vi "CAN test do RIO 3 tcpip.vi"() -> ()   [LabVIEW 2014]
doc: "This example demonstrates frame streaming output using an NI-Embedded CAN for RIO interface. \n\nThis example can run against any input example, assuming you have a properly terminated CAN cable connected to two CAN ports."
uses:
  <vilib>/Platform/TimedLoop/XDataNode/XDataNode.xnode
  <vilib>/Platform/TimedLoop/XDataNode/nitl_modes.ctl
  <vilib>/Platform/TimedLoop/XDataNode/XDNodeRunTimeDep.lvlib
  <vilib>/Platform/TimedLoop/XDataNode/wakeup.ctl
  <vilib>/Platform/TimedLoop/XDataNode/timing_clust.ctl
  <resource>/objmgr/RioEmbeddedCANInterface.rc
  <vilib>/Utility/Variable/NI_VariableUtilities.lvlib
  Data Communication/Network Streams/Simple Network Streams/support/Network Stream Command.ctl
  <vilib>/RioEmbeddedCAN/RioEmbeddedCAN.llb/CANFrameControl.ctl
  <vilib>/RioEmbeddedCAN/RioEmbeddedCAN.llb/CANWaitTransmitComplete.vi
  <vilib>/NI/STM/TCP/Get Connection Reference (TCP).vi
  <vilib>/NI/STM/TCP/Write Meta Data (TCP Ref).vi
  <vilib>/NI/STM/SubVIs/MetaDataElement.ctl
  <vilib>/NI/STM/TCP/Write Message (TCP).vi
panel:
  out "error out 2":errorcluster
  in  "stop 3":bool
  out "ilosc mesag":dbl
  out "data string":string
  out "Numeric":i32
  in  "stop 2":bool
  out "Waveform Chart 5":cluster{"mean":dbl, "output 3":u16}(graph)
  out "Waveform Chart 2":cluster{"rms value":dbl, "output 2":dbl}(graph)
  in  "odczyt 2":bool=TRUE
  out "Frames 2":string[][](table) caption="Frames"
  in  "Number of Frames to Display 2":i32=15
  in  "Hexadecimal? 2":bool
  out "error out":errorcluster
  out "x != y?":bool
  out "(hi.lo)":u16
  out "x .or. y?":bool
  out "data":T1[](array[typedef]) {"type" items=["CAN Data", "CAN Remote"]; "identifier" format="%.0x"}
  in  "stop":bool
  out "Variable2":bool
  in  "CAN frame 2":T1={"identifier"=2, "extended?"=FALSE, "type"=0, "payload"=[1, 2, 3, 4, 5, 6, 7, 8]} {"type" items=["CAN Data", "CAN Remote"]; "identifier" format="%.0x"}
  in  "Stop Button":bool
  in  "Write":bool
  in  "CAN frame":T1={"identifier"=2, "extended?"=FALSE, "type"=0, "payload"=[1, 2, 3, 4, 5, 6, 7, 8]} {"type" items=["CAN Data", "CAN Remote"]; "identifier" format="%.0x"}
  in  "receive queue size":u32=50
  in  "baud rate":u32=500000
  in  "interface index":u32
  # "Overview: Demonstrates frame streaming output using an NI-Embedded CAN for RIO interface.\nInstructions: Run the VI."
  # "See VI Info <Ctrl+I> for more information on how to use this example"
  # "Interface Configuration"
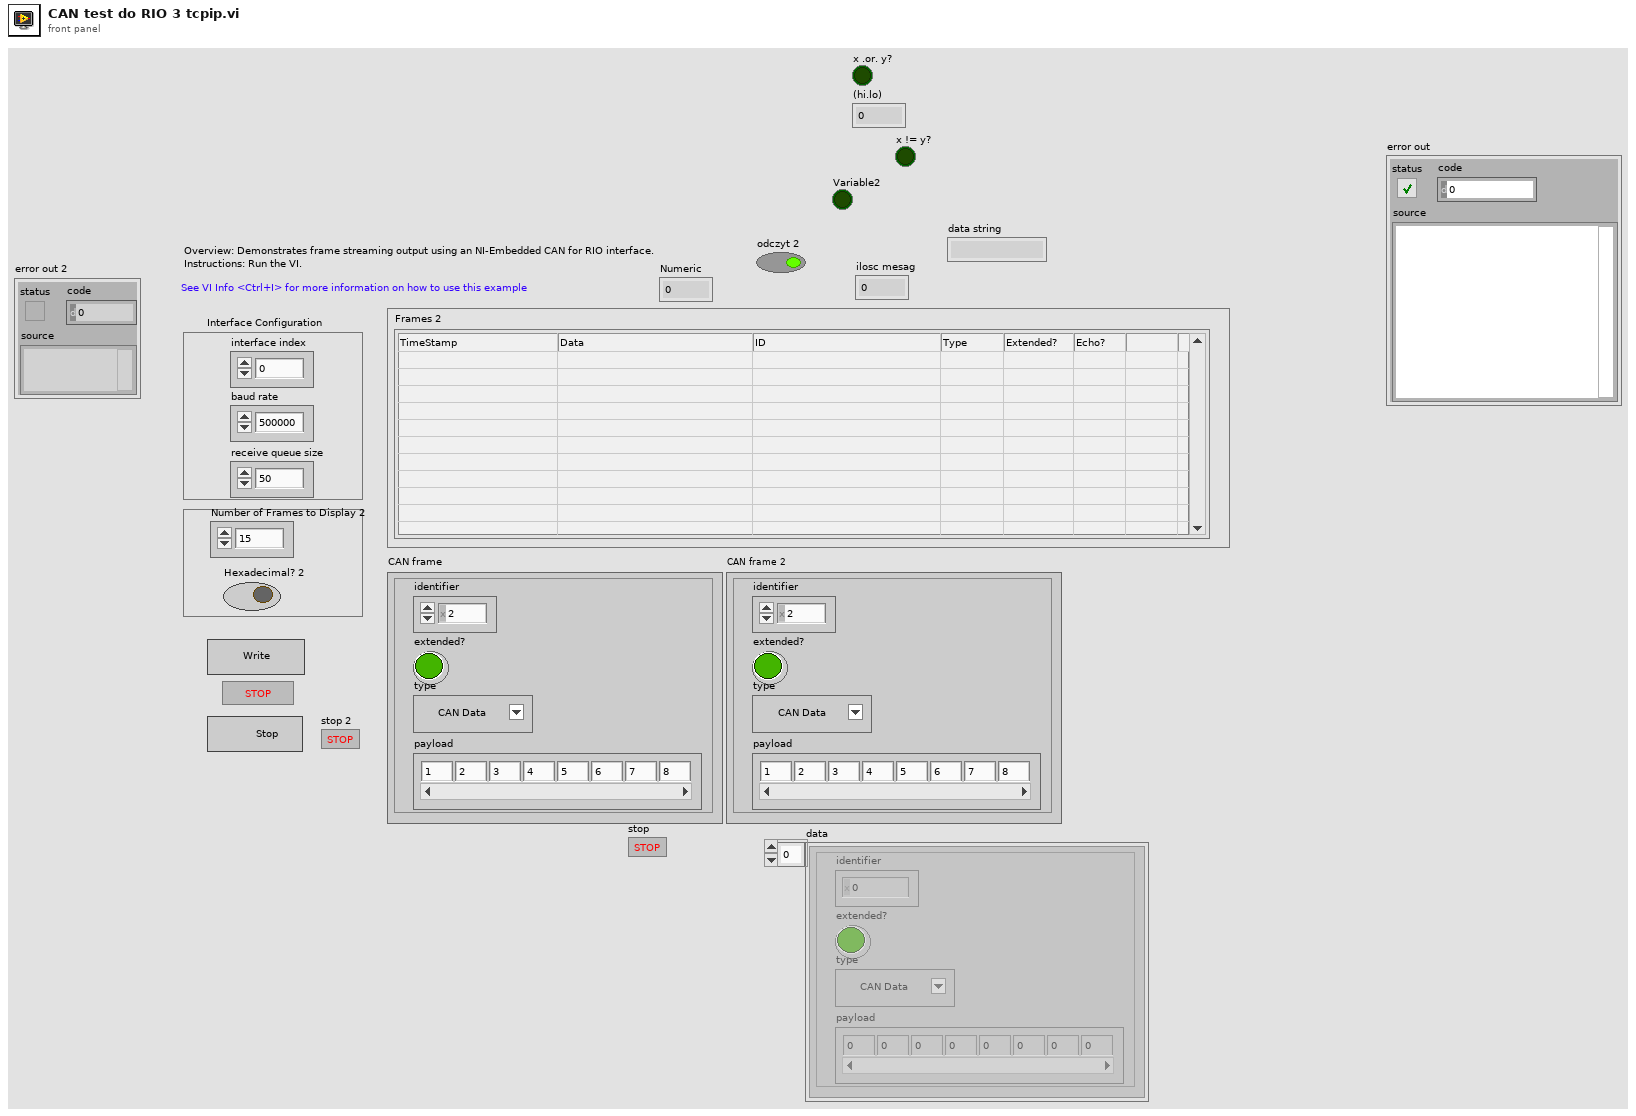
[diagram p1: front panel]
types:
  T1 = typedef "CANFrameControl.ctl" = cluster{"identifier":u32, "extended?":bool, "type":u8, "payload":u8[]}
  T2 = typedef "NI STM.lvlib/MetaDataElement.ctl" = string
  T3 = typedef "XDNodeRunTimeDep.lvlib/timing_clust.ctl" = cluster{"Expected End [f-1]":u64, "Actual End [f-1]":u64, "Finished Late? [f-1]":bool, "Expected End [i-1]":u64, "Actual End [i-1]":u64, "Finished Late? [i-1]":bool, "Expected Start [i]":u64, "Actual Start [i]":u64, "Expected Start [f]":u64, "Actual Start [f]":u64, "Source Name":string, "Structure Name":string, "Period":i64, "Deadline":i64, "Offset":i64, "Start":i64, "Priority":i32, "Timeout":i32, "Mode":T4, "Wakeup Reason":T5, "Error":errorcluster, "Source Type":string, "Secondary Source Type":string, "Global End Time":u64, "Global Start Time":u64, "Frame Duration":u64, "Iteration Duration":u64, "Assigned CPU":i32, "I/O Scan Engine Mode":u32}
  T4 = typedef "XDNodeRunTimeDep.lvlib/nitl_modes.ctl" = enum32{"No Change", "Process missed periods, maintain original phase", "Discard missed periods, maintain original phase", "Process missed periods, ignore original phase", "Discard missed periods, ignore original phase"}
  T5 = typedef "XDNodeRunTimeDep.lvlib/wakeup.ctl" = enum32{"Normal", "Aborted", "Asynchronous wakeup", "Timing source error", "Timed loop error", "Timeout"}
  T6 = cluster{"identifier":u32, "extended?":bool, "type":u8, "payload":u8[]}
  T7 = typedef "NI STM.lvlib/TCP Connection Info.ctl" = cluster{"connection ID":refnum<k5>, "meta data":T2[]}
  T8 = typedef "Network Stream Command.ctl" = cluster{"Message":string, "Message Data":variant}
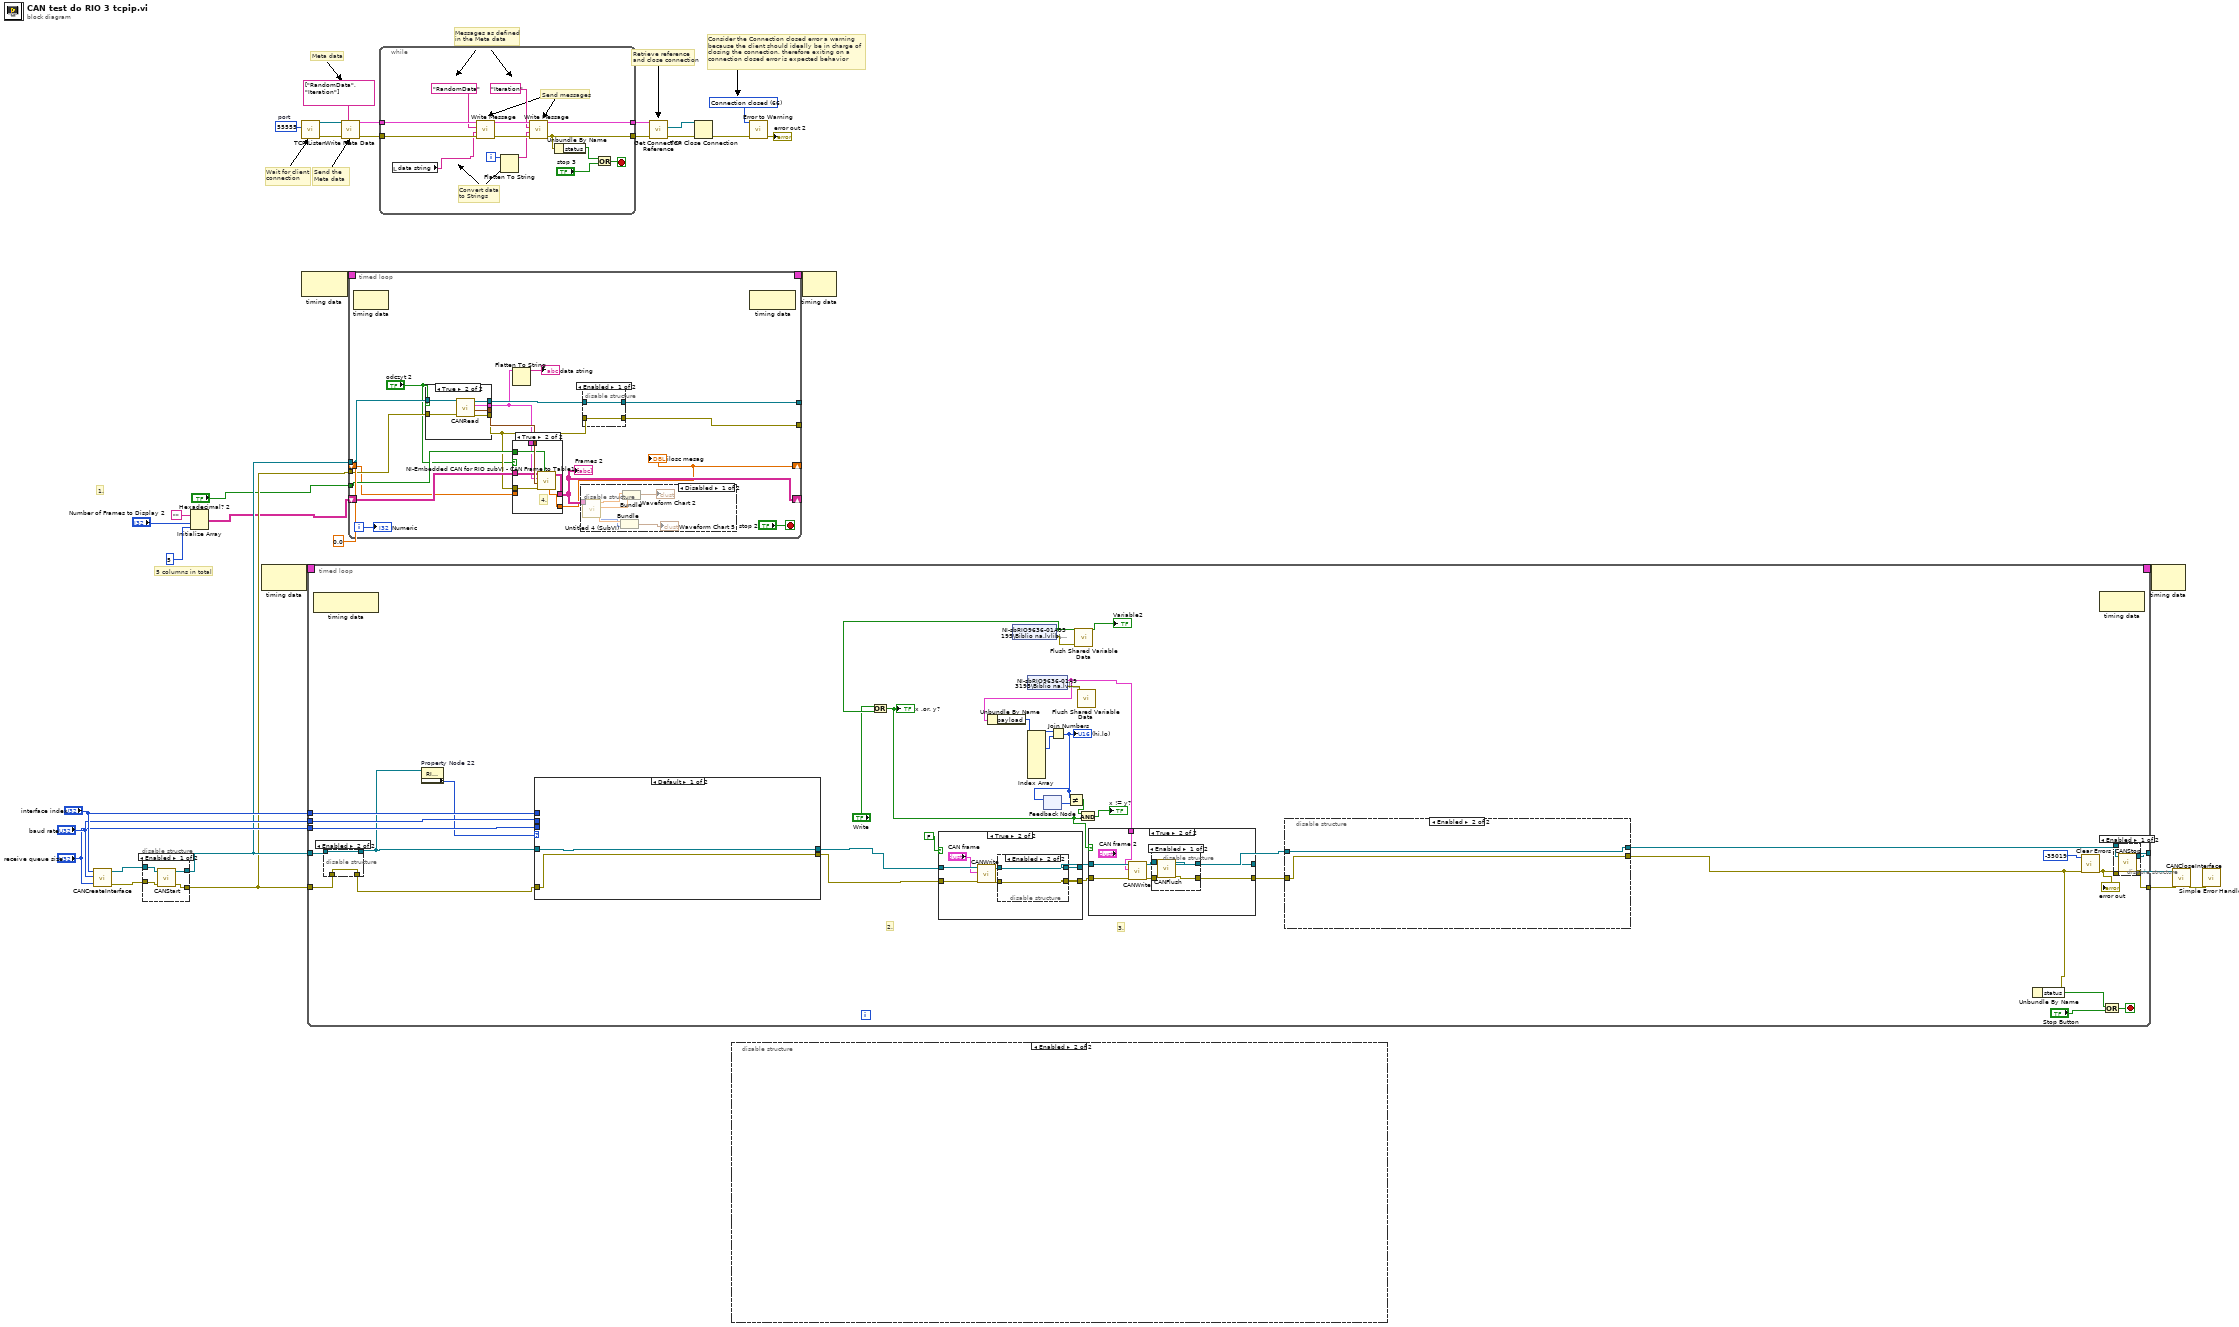
[diagram p0: block diagram]
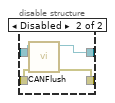
[diagram p4: hidden frame]
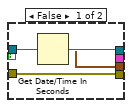
[diagram p5: hidden frame]
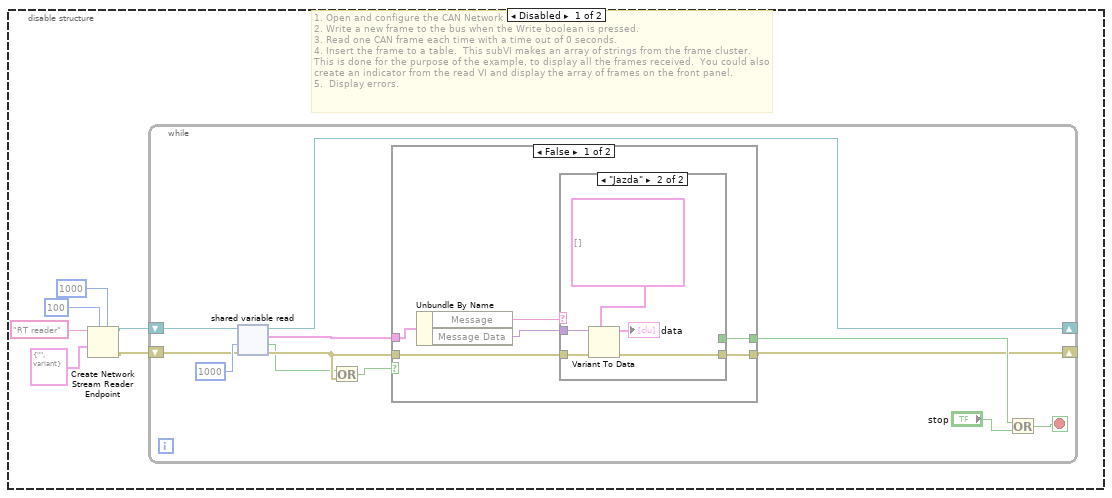
[diagram p7: hidden frame]
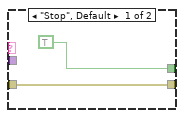
[diagram p8: hidden frame]
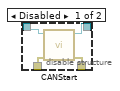
[diagram p10: hidden frame]
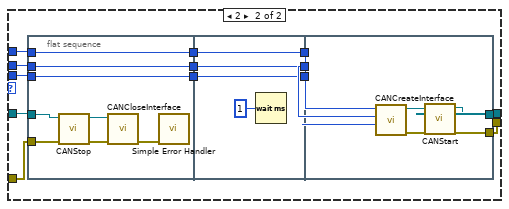
[diagram p12: hidden frame]
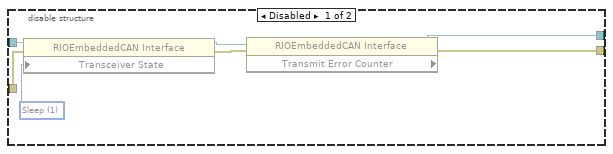
[diagram p13: hidden frame]
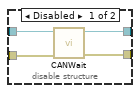
[diagram p17: hidden frame]
diagram:
  w10 = 66 items=["No Error", "Argument Error", "Memory Full", "Out of Zone", "End of File", "File Already Open", "Generic File IO Error", "File Not Found", "File Permission Error", "Disk Full", "Duplicate Path", "Too Many Files Open", "Not Enabled", "Resource File Not Found", "Cannot Add Resource", "Resource Not Found", "Image Not Found", "Image Memory Error", "Pen Does Not Exist", "Config Bad Type", "Config Token Not Found", "Config Parse Error", "Config Memory Error", "Bad External Code Format", "Bad External Code Offset", "External Code Not Present", "Null Window", "Destroy Window Mixup", "Null Menu", "Print Aborted", "Bad Print Record", "Print Driver Error", "Windows Error During Print", "Memory Error During Print", "Print Dialog Error", "Generic Print Error", "Invalid Device Refnum", "Device Not Found", "Device Parameter Error", "Device Unit Error", "Can't Open Device", "Device Call Aborted", "Generic Error", "Cancelled By User", "Object ID Too Low", "Object ID Too High", "Object Not In Heap", "Unknown Heap", "Bad DefProc ID", "DefProc Not In Table", "Message Out Of Range", "Null Method", "Unknown Message", "Manager Call Not Supported", "Bad address", "Connection In progress", "Connection timed out", "Connection is already in progress", "Network attribute not supported", "Network error", "Address in use", "System out of memory", "Connection aborted", "Connection refused", "Connection is not connected", "Connection is already connected", "Connection closed", "Initialize error (interapplication manager)", "Bad occurrence", "Wait on unbound occurrence handler", "Occurrence queue overflow", "Bad path", "Semaphore not signaled", "Unrecognized type (interapplication manager)"] ("1st Error to Convert")
  w1 = u16 55555  # port
  # "Consider the Connection closed error a warning because the client should ideally be in charge of closing the connection, therefore exiting on a connection closed error is expected behavior"
  # "Retrieve reference and close connection"
  # "Meta data"
  # "Messages as defined\nin the Meta data"
  # "Wait for client\nconnection"
  # "Send the\nMeta data"
  # "5 columns in total"
  # "1."
  n1 = call <vilib>:"CANCreateInterface.vi"("receive queue size (5)"="receive queue size", "baud rate (125000 bps)"="baud rate", "interface index"="interface index") -> ("error out"=w24:errorcluster, "interface object out"=w25:refnum<k20>)  [unwired: 7 in]
  n2 = disable-structure shown="Enabled" {
    disable-tunnel: w25 -> [w37 w39]
    disable-tunnel: [w36 w39] -> w21
    disable-tunnel: w24 -> [w35 w38]
    disable-tunnel: [w34 w38] -> w20
    frame Enabled {
      n3 = call <vilib>:"CANStart.vi"("error in (no error)"=w35, "interface object in"=w37) -> ("error out"=w34:errorcluster, "interface object out"=w36:refnum<k20>)  [unwired: 8 in]
    }
    frame Disabled {
    }
  }
  n4 = Initialize Array("" ("Empty String Constant"), "Number of Frames to Display 2", 5 ("dimension size")) -> (w16:string[][])
  n5 = node-c288 ("Input Node")() -> (w33:T3)  [unwired: 1 in]
  n6 = call <vilib>:"TCP Listen.vi"("port"=w1) -> ("error out"=w3:errorcluster, "connection ID"=w2:refnum<k5>)  [unwired: 3 in, 6 out]
  n7 = node-c288() -> (w23:T3)  [unwired: 1 in]
  n8 = timed-loop "Timed Loop" {
    timing: w33 -> [_]
    timing-out: [_] -> w32
    tunnel: w21 -> [w47]
    tunnel: w20 -> [w46]
    tunnel: [w50] -> w30
    tunnel: [w48] -> w29
    tunnel: "interface index" -> [w55]
    tunnel: "baud rate" -> [w54]
    tunnel: "receive queue size" -> [w53]
    stop <- w74 stop-if-true
    # "3."
    # "2."
    n9 = node-c288 ("Output Node")() -> ()  [unwired: 1 in, 1 out]
    n10 = disable-structure shown="Enabled" {
      disable-tunnel: w47 -> [w79 w80]
      disable-tunnel: [w78 w80] -> w41
      disable-tunnel: w46 -> [w77 w81]
      disable-tunnel: [w76 w81] -> w45
      frame Disabled {
        n11 = call <vilib>:"CANStart.vi"("error in (no error)"=w77, "interface object in"=w79) -> ("error out"=w76:errorcluster, "interface object out"=w78:refnum<k20>)  [unwired: 8 in]
      }
      frame Enabled {
      }
    }
    n12 = property on="Property Node 22" class="RIOEmbeddedCAN Interface"(reference=w41) -> ("Communication State"=w40:u32)  [unwired: 1 in, 2 out]
    n13 = case shown="Default" w40 {
      tunnel: [w88 w102] -> w56
      tunnel: w41 -> [w89 w98]
      tunnel: [w89 w96] -> w44
      tunnel: w55 -> [_ w101]
      tunnel: w54 -> [_ w100]
      tunnel: w53 -> [_ w99]
      tunnel: w45 -> [w88 w97]
      frame Default {
      }
      frame 2 {
        n14 = flat-sequence {
          tunnel: w98 -> [w106]
          tunnel: w99 -> [w108]
          tunnel: w100 -> [w109]
          tunnel: w101 -> [w110]
          tunnel: [w110] -> w95
          tunnel: [w109] -> w93
          tunnel: [w108] -> w91
          tunnel: w97 -> [w103]
          tunnel: w95 -> [w114]
          tunnel: [w114] -> w94
          tunnel: w93 -> [w113]
          tunnel: [w113] -> w92
          tunnel: w91 -> [w112]
          tunnel: [w112] -> w90
          tunnel: [w116] -> w102
          tunnel: [w117] -> w96
          tunnel: w94 -> [w121]
          tunnel: w92 -> [w120]
          tunnel: w90 -> [w119]
          frame #0 {
            n15 = call <vilib>:"CANStop.vi"("error in (no error)"=w103, "interface object in"=w106) -> ("error out"=w104:errorcluster, "interface object out"=w105:refnum<k20>)  [unwired: 8 in]
            n16 = call <vilib>:"CANCloseInterface.vi"("error in (no error)"=w104, "interface object in"=w105) -> ("error out"=w107:errorcluster)  [unwired: 9 in]
            n17 = call <vilib>:"Simple Error Handler.vi"("error in (no error)"=w107) -> ()  [unwired: 4 in, 5 out]
          }
          frame #1 {
            n18 = Wait (ms)(milliseconds to wait=u32 1) -> ()  [unwired: 1 out]
          }
          frame #2 {
            n19 = call <vilib>:"CANCreateInterface.vi"("receive queue size (5)"=w119, "baud rate (125000 bps)"=w120, "interface index"=w121) -> ("error out"=w115:errorcluster, "interface object out"=w118:refnum<k20>)  [unwired: 7 in]
            n20 = call <vilib>:"CANStart.vi"("error in (no error)"=w115, "interface object in"=w118) -> ("error out"=w116:errorcluster, "interface object out"=w117:refnum<k20>)  [unwired: 8 in]
          }
        }
      }
    }
    n21 = case shown="True" FALSE {
      tunnel: w44 -> [w147 w155]
      tunnel: w56 -> [w148 w154]
      tunnel: [w147 w152] -> w66
      tunnel: [w148 w151] -> w69
      frame False {
      }
      frame True {
        n22 = call <vilib>:"CANWrite.vi"("error in (no error)"=w154, "CAN frame"="CAN frame", "interface object in"=w155) -> ("error out"=w150:errorcluster, "interface object out"=w153:refnum<k20>)  [unwired: 7 in]
        n23 = disable-structure shown="Enabled" {
          disable-tunnel: w153 -> [w159 w161]
          disable-tunnel: [w158 w161] -> w152
          disable-tunnel: [w157 w160] -> w151
          disable-tunnel: w150 -> [w156 w160]
          frame Disabled {
            n24 = call-poly <vilib>:"CANWait.vi"("error in (no error)"=w156, "interface object in"=w159) -> ("error out"=w157:errorcluster, "interface object out"=w158:refnum<k20>)  [unwired: 8 in]
          }
          frame Enabled {
          }
        }
      }
    }
    n25 = shared-variable "NI-sbRIO9636-01A93195\\Biblio na.lvlib\\status"() -> (w71:bool, error out=w72:errorcluster)  [unwired: 1 in]
    "Variable2" <- w71
    n26 = Or(x="Write", y=w71) -> (x .or. y?=w52:bool)
    "x .or. y?" <- w52
    n27 = shared-variable "NI-sbRIO9636-01A93195\\Biblio na.lvlib\\can1"() -> (w59:T6, error out=w68:errorcluster)  [unwired: 1 in]
    n28 = Unbundle By Name(w59) -> ("payload"=w64:u8[])
    n29 = Index Array(array=w64) -> (element #1=w62:u8, element #2=w63:u8)  [unwired: 8 in, 6 out]
    n30 = feedback #1() -> (w60:u16)  [unwired: 1 in]
    n31 = Join Numbers(hi=w62, lo=w63) -> ((hi.lo)=w61:u16)
    "(hi.lo)" <- w61
    n32 = feedback-in #1(w61) -> ()
    n33 = Not Equal?(x=w61, y=w60) -> (x != y?=w58:bool)
    n34 = call <vilib>:"Flush Shared Variable Data.vi"("error in (no error)"=w72) -> ()  [unwired: 10 in, 1 out]
    n35 = call <vilib>:"Flush Shared Variable Data.vi"("error in (no error)"=w68) -> ()  [unwired: 10 in, 1 out]
    n36 = And(x=w58, y=w52) -> (x .and. y?=→"x != y?":bool)
    n37 = case shown="True" w52 {
      tunnel: w69 -> [w133 w136]
      tunnel: [w132 w135] -> _
      tunnel: [w133 w134] -> w65
      tunnel: w66 -> [w132 w137]
      tunnel: w59 -> [_ w138]
      frame False {
      }
      frame True {
        n38 = call <vilib>:"CANWrite.vi"("error in (no error)"=w136, "CAN frame"=w138, "interface object in"=w137) -> ("error out"=w139:errorcluster, "interface object out"=w140:refnum<k20>)  [unwired: 7 in]
        n39 = disable-structure shown="Enabled" {
          disable-tunnel: w140 -> [w144 w146]
          disable-tunnel: w139 -> [w143 w145]
          disable-tunnel: [w142 w146] -> w135
          disable-tunnel: [w141 w145] -> w134
          frame Enabled {
            n40 = call <vilib>:"CANFlush.vi"("error in (no error)"=w143, "interface object in"=w144) -> ("error out"=w141:errorcluster, "interface object out"=w142:refnum<k20>)  [unwired: 8 in]
          }
          frame Disabled {
          }
        }
      }
    }
    n41 = disable-structure shown="Enabled" {
      disable-tunnel: w66 -> [w129 w131]
      disable-tunnel: w65 -> [w127 w130]
      disable-tunnel: [w123 w131] -> w43
      disable-tunnel: [w122 w130] -> w42
      frame Disabled {
        w128 = u32 1 items=["Normal", "Sleep"] ("Transceiver State")
        n42 = property class="RIOEmbeddedCAN Interface"(reference=w129, error in=w127, "Transceiver State"=w128) -> (reference out=w125:refnum<k20>, error out=w124:errorcluster)
        n43 = property class="RIOEmbeddedCAN Interface"(reference=w125, error in=w124) -> (reference out=w123:refnum<k20>, error out=w122:errorcluster, "Transmit Error Counter"=w126:u8)
      }
      frame Enabled {
      }
    }
    n44 = Unbundle By Name(w42) -> ("status"=w75:bool)
    n45 = call <vilib>:"Clear Errors.vi"("error in (no error)"=w42, "specific error code to clear (0: all)"=-35019) -> ("error out"=w49:errorcluster)  [unwired: 4 in, 1 out]
    "error out" <- w49
    n46 = node-c288 ("Input Node")() -> ()  [unwired: 1 in, 1 out]
    n47 = Or(x=w75, y="Stop Button") -> (x .or. y?=w74:bool)
    n48 = disable-structure shown="Enabled" {
      disable-tunnel: w43 -> [w85 w87]
      disable-tunnel: [w84 w87] -> w50
      disable-tunnel: w49 -> [w83 w86]
      disable-tunnel: [w82 w86] -> w48
      frame Enabled {
        n49 = call <vilib>:"CANStop.vi"("error in (no error)"=w83, "interface object in"=w85) -> ("error out"=w82:errorcluster, "interface object out"=w84:refnum<k20>)  [unwired: 8 in]
      }
      frame Disabled {
      }
    }
  }
  n50 = call-poly <vilib>:"Write Meta Data.vi"("meta data"=T2[] ["RandomData", "Iteration"] ("Meta data"), "error in"=w3, "connection ID"=w2) -> ("error out"=w5:errorcluster, "connection info out"=w4:T7)  [unwired: 2 in, 5 out]
  n51 = timed-loop {
    timing: w23 -> [_]
    timing-out: [_] -> w22
    tunnel: [w178] -> _
    tunnel: w21 -> [w178]
    tunnel: w20 -> [w177]
    shift-right: [w173] -> _
    shift-left: w16 -> [w174]
    tunnel: "Hexadecimal? 2" -> [w179]
    tunnel: [w176] -> _
    tunnel: [w175] -> _
    shift-right: [w165] -> _
    shift-left: 0.0 ("Numeric") -> [w164]
    i -> [w168]
    stop <- "stop 2" stop-if-true
    n52 = node-c288() -> ()  [unwired: 1 in, 1 out]
    n53 = case shown="True" "odczyt 2" {
      tunnel: w178 -> [w205 w212]
      tunnel: w177 -> [w206 w211]
      tunnel: [w204 w210] -> w180
      tunnel: [w206 w209] -> w170
      tunnel: [_ w208] -> w166
      tunnel: [w205 w207] -> w171
      frame False {
        n54 = Get Date/Time In Seconds() -> (seconds since 1Jan1904=w204:timestamp)
      }
      frame True {
        n55 = call <vilib>:"CANRead.vi"("error in (no error)"=w211, "interface object in"=w212) -> ("error out"=w209:errorcluster, "timestamp"=w210:timestamp, "CAN frame"=w208:T1, "interface object out"=w207:refnum<k20>)  [unwired: 6 in]
      }
    }
    n56 = Flatten To String(anything=w166) -> (data string=→"data string":string)  [unwired: 3 in, 2 out]
    n57 = case shown="True" "odczyt 2" {
      tunnel: w180 -> [_ w197]
      tunnel: w179 -> [_ w196]
      tunnel: w174 -> [w189 w195]
      tunnel: [w189 w194] -> w173
      tunnel: w170 -> [_ w193]
      tunnel: w166 -> [_ w192]
      tunnel: [w188 w191] -> w165
      tunnel: w164 -> [w188 w190]
      frame False {
      }
      frame True {
        # "4."
        n58 = call "NI-Embedded CAN for RIO subVI - CAN Frame to Table1.vi"("ramki"=w190, "Hexadecimal?"=w196, "error in (no error)"=w193, "timestamp"=w197, "CAN frame"=w192, "Input Array"=w195) -> ("Output Array"=w194:string[][], "ilosc mesagy"=w191:dbl)  [unwired: 2 in, 2 out]
      }
    }
    "Frames 2" <- w173
    "ilosc mesag" <- w165
    n59 = disable-structure shown="Disabled" {
      disable-tunnel: w173 -> [w181 _]
      frame Disabled {
        n60 = call "Untitled 4 (SubVI).vi"("Output Array"=w181) -> ("mean"=w187:dbl, "output 3"=w186:u16, "output 2"=w184:dbl, "rms value"=w185:dbl)  [unwired: 4 in, 3 out]
        n61 = Bundle("mean"=w187, "output 3"=w186) -> (→"Waveform Chart 5":cluster{"mean":dbl, "output 3":u16})  [unwired: 1 in]
        n62 = Bundle("rms value"=w185, "output 2"=w184) -> (→"Waveform Chart 2":cluster{"rms value":dbl, "output 2":dbl})  [unwired: 1 in]
      }
      frame Enabled {
      }
    }
    n63 = disable-structure shown="Enabled" {
      disable-tunnel: [w199 w201] -> w175
      disable-tunnel: [w198 w200] -> w176
      disable-tunnel: w170 -> [w198 w202]
      disable-tunnel: w171 -> [w199 w203]
      frame Enabled {
      }
      frame Disabled {
        n64 = call <vilib>:"CANFlush.vi"("error in (no error)"=w202, "interface object in"=w203) -> ("error out"=w200:errorcluster, "interface object out"=w201:refnum<k20>)  [unwired: 8 in]
      }
    }
    n65 = node-c288() -> ()  [unwired: 1 in, 1 out]
    "Numeric" <- w168
  }
  n66 = while {
    tunnel: w4 -> [w228]
    tunnel: w5 -> [w227]
    tunnel: [w226] -> w6
    tunnel: [w220] -> w8
    i -> [w217]
    stop <- w221 stop-if-true
    # "Send messages"
    # "Convert data\nto Strings"
    n67 = local read "data string"() -> (w215:string)
    n68 = call-poly <vilib>:"Write Message.vi"("error in"=w227, "data"=w215, "name"="RandomData" ("Name"), "connection info in"=w228) -> ("error out"=w225:errorcluster, "connection info out"=w224:T7)  [unwired: 1 in, 5 out]
    n69 = Flatten To String(anything=w217) -> (data string=w216:string)  [unwired: 1 in, 4 out]
    n70 = call-poly <vilib>:"Write Message.vi"("error in"=w225, "data"=w216, "name"="Iteration" ("Name"), "connection info in"=w224) -> ("error out"=w220:errorcluster, "connection info out"=w226:T7)  [unwired: 1 in, 5 out]
    n71 = Unbundle By Name(w220) -> ("status"=w219:bool)
    n72 = Or(x=w219, y="stop 3") -> (x .or. y?=w221:bool)
  }
  n73 = call-poly <vilib>:"Get Connection Reference.vi"("error in"=w8, "connection info in"=w6) -> ("error out"=w9:errorcluster, "connection ID out"=w7:refnum<k5>)  [unwired: 8 out]
  n74 = TCP Close Connection(connection ID=w7, error in (no error)=w9) -> (error out=w11:errorcluster)  [unwired: 2 out]
  n75 = disable-structure shown="Enabled" {
    frame Disabled {
      # "1. Open and configure the CAN Network Interface.\n2. Write a new frame to the bus when the Write boolean is pressed.\n3. Read one CAN frame each time with a time out of 0 seconds.\n4. Insert the frame to a table.  This subVI makes an array of strings from the frame cluster.  This is done for the purpose of the example, to display all the frames received.  You could also create an indicator from the read VI and display the array of frames on the front panel. \n5.  Display errors."
      n76 = Create Network Stream Reader Endpoint(5:1000 ("timeout in ms (-1)"), 7:100 ("reader buffer size"), 9:T8 {"Message"="", "Message Data"=variant} ("Message Cluster"), 11:"RT reader" ("reader url")) -> (0:w230:errorcluster, 3:w231:refnum<k21>)  [unwired: 3 in]
      n77 = while {
        shift-right: [w235] -> _
        shift-left: w231 -> [w245]
        shift-right: [w236] -> _
        shift-left: w230 -> [w244]
        stop <- w238 stop-if-true
        n78 = shared-variable-read(w245, w244, 1000 ("timeout ms")) -> (w235:refnum<k21>, w241:errorcluster, w240:bool, w243:T8)
        n79 = Or(x=w240, y=w241) -> (x .or. y?=w242:bool)
        n80 = case shown="False" w242 {
          tunnel: w241 -> [w252 w260]
          tunnel: [w251 w260] -> w236
          tunnel: [w250 _] -> w237
          tunnel: w243 -> [w249 _]
          frame False {
            n81 = Unbundle By Name(w249) -> ("Message"=w248:string, "Message Data"=w247:variant)
            n82 = case shown="\"Jazda\"" w248 {
              tunnel: w252 -> [w254 w259]
              tunnel: [w254 w258] -> w251
              tunnel: [TRUE _] -> w250
              tunnel: w247 -> [_ w257]
              frame "Stop", Default {
              }
              frame "Jazda" {
                n83 = Variant To Data(error in=w259, type=T1[] [], Variant=w257) -> (data=→"data":T1[], error out=w258:errorcluster)
              }
            }
          }
          frame True {
          }
        }
        n84 = Or(x=w237, y="stop") -> (x .or. y?=w238:bool)
      }
    }
    frame Enabled {
    }
  }
  n85 = call <vilib>:"Error to Warning.vi"("1st Error to Convert"=w10, "error in"=w11) -> ("warning out"=→"error out 2":errorcluster)  [unwired: 3 in, 10 out]
  n86 = node-c288(w22) -> ()  [unwired: 1 out]
  n87 = node-c288 ("Output Node")(w32) -> ()  [unwired: 1 out]
  n88 = call <vilib>:"CANCloseInterface.vi"("error in (no error)"=w29, "interface object in"=w30) -> ("error out"=w31:errorcluster)  [unwired: 9 in]
  n89 = call <vilib>:"Simple Error Handler.vi"("error in (no error)"=w31) -> ()  [unwired: 4 in, 5 out]
